vi "SEQ Reset sequencer.vi"(8 "error in":errorcluster, 11 "Refnum in":refnum<k20>) -> (0 "error out":errorcluster, 3 "Refnum out":T1)   [LabVIEW 2019, in "FPGA sequencer API.lvlib"]
uses:
  FPGA sequencer API.lvlib
  FPGA sequencer ref.ctl
  f3d39e56-424e-4e37-9b38-d23f2d74d210.vi
  <vilib>/Utility/error.llb/Error Cluster From Error Code.vi
  <vilib>/rvi/errors/niLvFpgaAdjustHostInterfaceError.vi
  <vilib>/rvi/interface/nirviReadWriteControl/nirviReadWriteControl.xnode
  NiFpgaLv.dll
  <vilib>/rvi/interface/Simulation/niFpgaSimulationCallBeginRW.vi
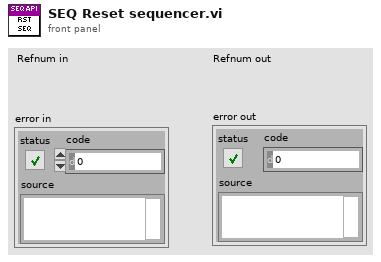
[diagram p1: front panel]
types:
  T1 = typedef "FPGA sequencer API.lvlib/FPGA sequencer ref.ctl" = refnum<k20>
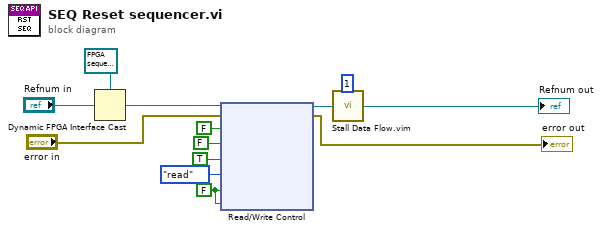
[diagram p0: block diagram]
diagram:
  w1 = FALSE ("seq.start")
  n1 = Dynamic FPGA Interface Cast(Session In=T1 refnum ("FPGA VI Reference Out"), Type="Refnum in") -> (Session Out=w11:T1)
  n2 = xnode "Read/Write Control"("FPGA VI Reference In"=w11, "error in"="error in", "seq.continous"=FALSE, "seq.rst"=FALSE, "seq.rst"=TRUE, "memo mode"=enum16{"flush", "reset", "write", "read"}."read" ("dram mode"), "seq.start"=w1, "gen.enable"=w1) -> ("FPGA VI Reference Out"=w6:T1, "error out"=→"error out":errorcluster)
  n3 = call "Stall Data Flow.vim"("value in"=w6, "milliseconds to wait"=u32 1) -> ("value out"=→"Refnum out":T1)  [unwired: 1 out]
